vi "3) Group Subscription.vi"() -> ()   [LabVIEW 2020, in "VectoScratch.lvlib"]
uses:
  VectoScratch.lvlib
  Vecto/Group Info.ctl
  Vecto/Publish Config.ctl
  Vecto/Group Data Type.ctl
  Vecto/Channel Init.ctl
  Vecto/Group/Group.lvclass
  C:/dev/lv20CE/relink/lv-vecto/Vecto/GroupAbstract/GroupAbstract.lvclass
  Vecto/ChannelService/Create Group Abstract.vi
  Vecto/ChannelService/ChannelService.lvclass
  VectoConfig/VectoConfig.lvlib
  Vecto/Group Config/Group Config.lvclass
  Vecto/RemoteDataService/RemoteDataService.lvclass
  Vecto/SequenceCountService/SequenceCountService.lvclass
panel:
  out "Timestamp":dbl format="%<%H:%M:%S%3u>T"
  out "Chart":dbl[][](graph)
  out "error out":errorcluster
  out "i":i32
  in  "stop":bool
  in  "Publish Address":string="230.0.0.100"
  in  "Publish Port":u16=20000
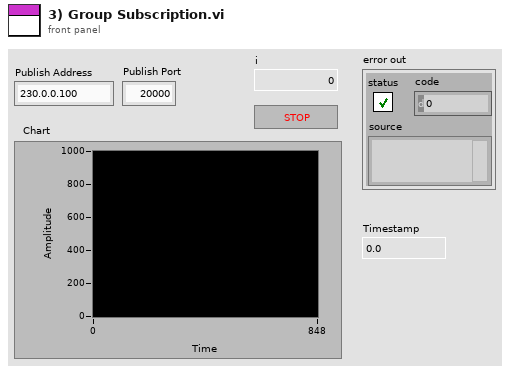
[diagram p1: front panel]
types:
  T1 = typedef "VectoConfig.lvlib/Group Data Type.ctl" = enum16{"Double", "String"}
  T2 = typedef "VectoConfig.lvlib/Publish Config.ctl" = cluster{"Address":string, "Port":u16}
  T3 = typedef "VectoConfig.lvlib/Group Info.ctl" = cluster{"System":string, "Cluster":string, "Node":string, "Task":string, "Name":string}
  T4 = typedef "VectoConfig.lvlib/Channel Init.ctl" = cluster{"Name":string, "Resource":string}
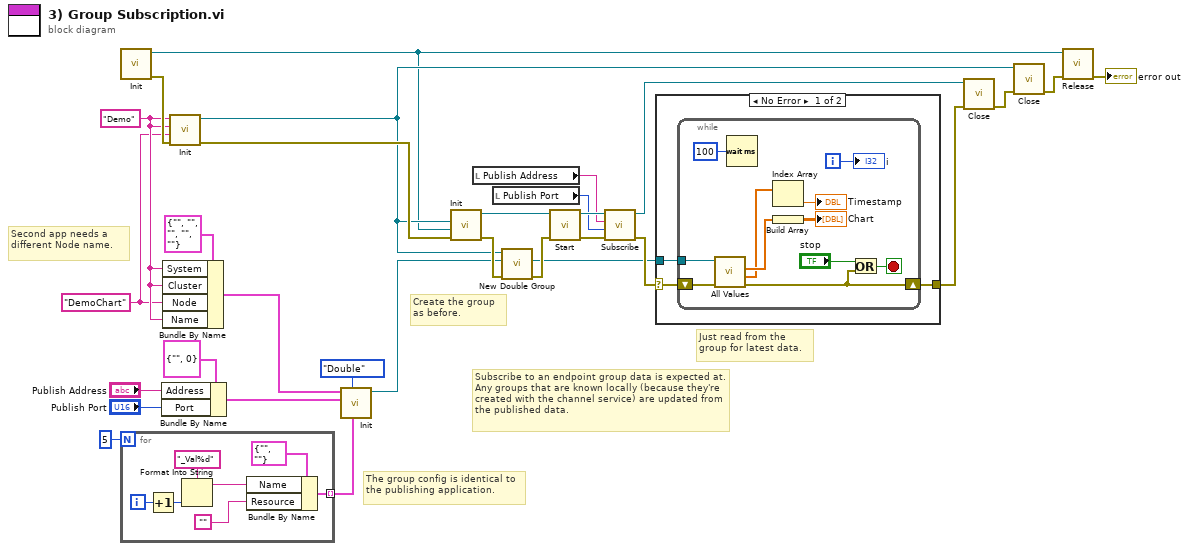
[diagram p0: block diagram]
diagram:
  w1 = "DemoChart" ("Node")
  w10 = "Demo" ("System")
  # "The group config is identical to the publishing application."
  # "Second app needs a different Node name."
  # "Just read from the group for latest data."
  # "Subscribe to an endpoint group data is expected at. Any groups that are known locally (because they're created with the channel service) are updated from the published data."
  # "Create the group as before."
  n1 = call "Init.vi"() -> ("error out"=w26:errorcluster, "SequenceCountService out"=w17:refnum<class "SequenceCountService.lvclass">)  [unwired: 10 in]
  n2 = for {
    N: 5 -> [_]
    tunnel: [w32] -> w11 mode=indexing
    i -> [w37]
    n3 = Increment(x=w37) -> (x+1=w36:i32)
    n4 = Format Into String(format string="_Val%d", w36) -> (resulting string=w34:string)  [unwired: 2 in, 1 out]
    n5 = Bundle By Name(cluster=T4 {"Name"="", "Resource"=""} ("Channel Init"), "Name"=w34, "Resource"="") -> (w32:T4)
  }
  n6 = Bundle By Name(cluster=T2 {"Address"="", "Port"=0} ("Publish Config"), "Address"="Publish Address", "Port"="Publish Port") -> (w12:T2)
  n7 = Bundle By Name(cluster=T3 {"System"="", "Cluster"="", "Node"="", "Task"="", "Name"=""} ("Group Info"), "System"=w10, "Cluster"=w10, "Node"=w1, "Name"=w10) -> (w13:T3)
  n8 = call "Init.vi"("error in (no error)"=w26, "Node"=w1, "Cluster"=w10, "System"=w10) -> ("error out"=w27:errorcluster, "ChannelService out"=w19:refnum<class "ChannelService.lvclass">)  [unwired: 6 in]
  n9 = call "Init.vi"("Channels"=w11, "Group Data Type"=Group_Data_Type."Double", "Publish Config (None)"=w12, "Group Info"=w13) -> ("Group Config out"=w23:refnum<class "Group Config.lvclass">)  [unwired: 6 in, 1 out]
  n10 = call "Init.vi"("error in (no error)"=w27, "SequenceCountService"=w17, "ChannelService"=w19) -> ("error out"=w28:errorcluster, "RemoteDataService out"=w7:refnum<class "RemoteDataService.lvclass">)  [unwired: 7 in]
  n11 = local read "Publish Address"() -> (w4:string)
  n12 = local read "Publish Port"() -> (w3:u16)
  n13 = call "New Double Group.vi"("error in (no error)"=w28, "Group Config"=w23, "ChannelService in"=w19) -> ("error out"=w29:errorcluster, "Group"=w22:refnum<class "Group.lvclass">)  [unwired: 6 in, 1 out]
  n14 = call "Start.vi"("error in (no error)"=w29, "RemoteDataService in"=w7) -> ("error out"=w6:errorcluster, "RemoteDataService out"=w5:refnum<class "RemoteDataService.lvclass">)  [unwired: 8 in]
  n15 = call "Subscribe.vi"("error in (no error)"=w6, "Multicast Port"=w3, "Multicast Address"=w4, "RemoteDataService in"=w5) -> ("error out"=w30:errorcluster, "RemoteDataService out"=w2:refnum<class "RemoteDataService.lvclass">)  [unwired: 6 in]
  n16 = case shown="No Error" w30 {
    selector: w30 -> [w38 w52]
    tunnel: [w40 w52] -> w21
    tunnel: w22 -> [w39 _]
    frame No Error {
      n17 = while {
        shift-right: [w51] -> w40
        shift-left: w38 -> [w46]
        tunnel: w39 -> [w47]
        i -> [w48]
        stop <- w49 stop-if-true
        n18 = call "All Values.vi"("error in (no error)"=w46, "Group in"=w47) -> ("error out"=w51:errorcluster, "Timestamp"=w43:dbl[], "Scaled"=w44:dbl[])  [unwired: 5 in, 2 out]
        n19 = Wait (ms)(milliseconds to wait=u32 100) -> ()  [unwired: 1 out]
        n20 = Index Array(array=w43) -> (element=→"Timestamp":dbl)  [unwired: 1 in]
        n21 = Build Array(w44) -> (→"Chart":dbl[][])
        n22 = Or(x="stop", y=w51) -> (x .or. y?=w49:bool)
        "i" <- w48
      }
    }
    frame Error {
    }
  }
  n23 = call "Close.vi"("error in (no error)"=w21, "RemoteDataService in"=w2) -> ("error out"=w20:errorcluster)  [unwired: 9 in]
  n24 = call "Close.vi"("error in (no error)"=w20, "ChannelService in"=w19) -> ("error out"=w18:errorcluster)  [unwired: 9 in]
  n25 = call "Release.vi"("error in (no error)"=w18, "SequenceCountService in"=w17) -> ("error out"=→"error out":errorcluster)  [unwired: 9 in]
